vi "그림전송실험서버.vi"() -> ()   [LabVIEW 2018]
panel:
  in  "파일 경로(대화 상자 사용)":path
  out "All Files in Dir":path[](array[path]) caption="디렉토리내의 모든 파일"
  in  "Folder Path":path caption="폴더 경로"
  in  "정지":bool
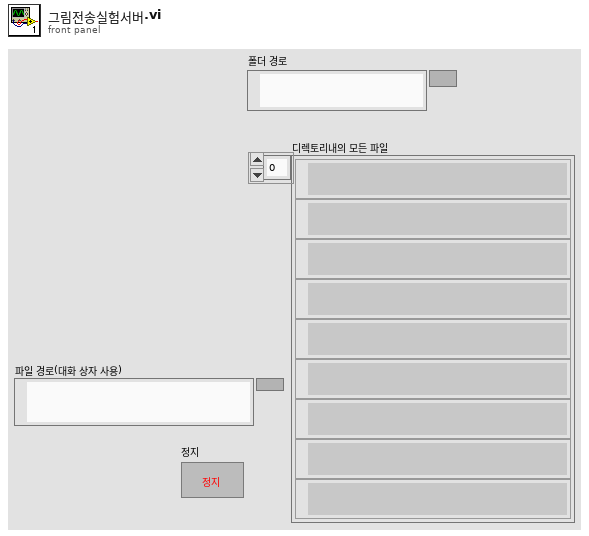
[diagram p1: front panel]
types:
  T1 = enum16{"open", "replace", "create", "open or create", "replace or create", "replace or create with confirmation"}
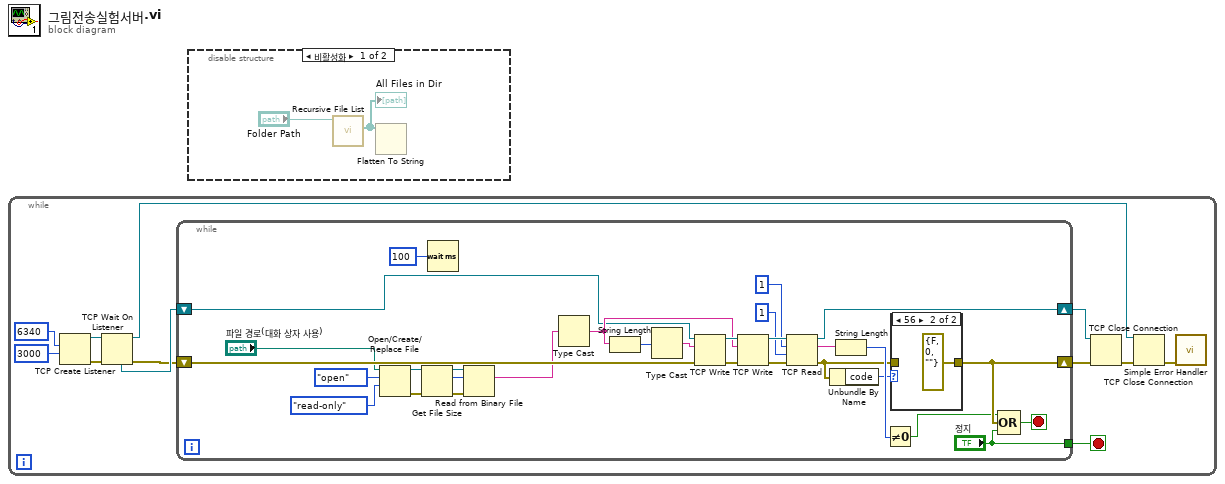
[diagram p0: block diagram]
diagram:
  n1 = while {
    stop <- w3 stop-if-true
    n2 = TCP Create Listener(9:3000 ("타임아웃 ms (25000)"), 10:u16 6340 ("포트")) -> (0:w9:errorcluster, 3:w12:refnum<k5>)  [unwired: 3 in, 1 out]
    n3 = TCP Wait On Listener(8:w9, 11:w12) -> (0:w5:errorcluster, 3:w1:refnum<k5>, 4:w7:refnum<k5>)  [unwired: 2 in, 2 out]
    n4 = while {
      shift-right: [w29] -> w6
      shift-left: w7 -> [w30]
      shift-right: [w24] -> w4
      shift-left: w5 -> [w28]
      tunnel: ["정지"] -> w3
      stop <- w25 stop-if-true
      n5 = Open/Create/Replace File(file path (use dialog)="파일 경로(대화 상자 사용)", operation (0:open)=T1."open" ("동작(0:open)"), access (0:read/write)=enum16{"read/write", "read-only", "write-only"}."read-only" ("접근(0:읽기/쓰기)")) -> (refnum out=w17:refnum<file>, error out=w19:errorcluster)  [unwired: 3 in, 1 out]
      n6 = Get File Size(file=w17, error in=w19) -> (refnum out=w18:refnum<file>, size (in bytes)=w21:i64, 0:w20:errorcluster)
      n7 = Wait (ms)(milliseconds to wait=u32 100 ("대기 시간 (ms)")) -> ()  [unwired: 1 out]
      n8 = Read from Binary File(8:w20, 10:w21, 11:w18) -> (2:w13:string)  [unwired: 3 in, 3 out]
      n9 = Type Cast(x=w13) -> (*(type *) &x=w37:string)  [unwired: 1 in]
      n10 = String Length(string=w37) -> (length=w36:i32)
      n11 = Type Cast(x=w36) -> (*(type *) &x=w35:string)  [unwired: 1 in]
      n12 = TCP Write(connection ID=w30, data in=w35, error in (no error)=w28) -> (connection ID out=w39:refnum<k5>, error out=w38:errorcluster)  [unwired: 1 in, 1 out]
      n13 = TCP Write(connection ID=w39, data in=w37, error in (no error)=w38) -> (connection ID out=w40:refnum<k5>, error out=w41:errorcluster)  [unwired: 1 in, 1 out]
      n14 = TCP Read(connection ID=w40, bytes to read=1 ("읽을 바이트"), error in (no error)=w41, 9:1 ("타임아웃 ms (25000)")) -> (connection ID out=w29:refnum<k5>, data out=w32:string, error out=w26:errorcluster)  [unwired: 1 in]
      n15 = Unbundle By Name(w26) -> ("code"=w27:i32)
      n16 = String Length(string=w32) -> (length=w31:i32)
      n17 = Not Equal To 0?(x=w31) -> (x != 0?=w23:bool)
      n18 = case shown="56" w27 {
        tunnel: w26 -> [w43 _]
        tunnel: [w43 errorcluster {"status"=FALSE, "code"=0, "source"=""} ("에러 상수")] -> w24
        frame Default {
        }
        frame 56 {
        }
      }
      n19 = Compound Arithmetic op=OR(w23, w24, "정지") -> (w25:bool)
    }
    n20 = TCP Close Connection(connection ID=w6, error in (no error)=w4) -> (error out=w8:errorcluster)  [unwired: 1 in, 1 out]
    n21 = TCP Close Connection(connection ID=w1, error in (no error)=w8) -> (error out=w2:errorcluster)  [unwired: 1 in, 1 out]
    n22 = call <vilib>:"Simple Error Handler.vi"("error in (no error)"=w2) -> ()  [unwired: 4 in, 5 out]
  }
  n23 = disable-structure shown="비활성화" {
    frame Disabled {
      n24 = call <vilib>:"Recursive File List.vi"("Folder Path"="Folder Path") -> ("All Files in Dir"=w46:path[])  [unwired: 6 in, 4 out]
      "All Files in Dir" <- w46
      n25 = Flatten To String(anything=w46) -> ()  [unwired: 3 in, 3 out]
    }
    frame Enabled {
    }
  }
